vi "GetSop.vi"(8 "error in (no error)":errorcluster, 11 "ModbusSp in":refnum<class "ModbusSp.lvclass">) -> (0 "error out":errorcluster, 2 "value":bool, 3 "ModbusSp out":refnum<class "ModbusSp.lvclass">)   [LabVIEW 2019, in "ModbusSp.lvclass"]
uses:
  ModbusSp.lvclass
  ModbusSp.lvclass/ModbusSp.ctl
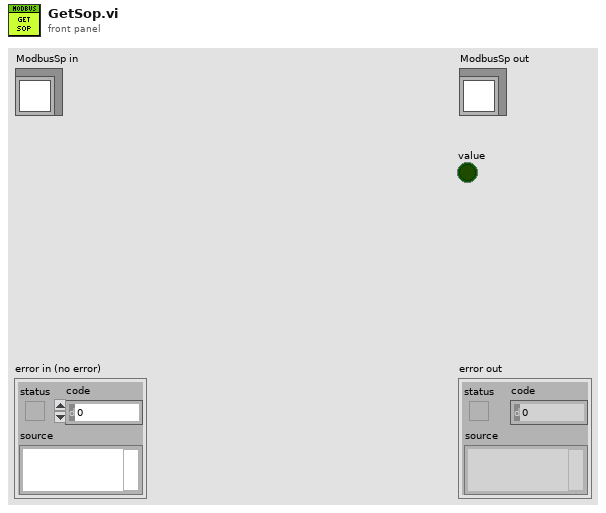
[diagram p1: front panel]
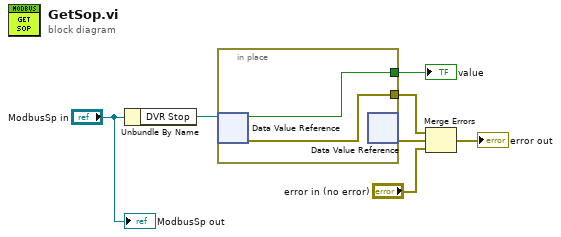
[diagram p0: block diagram]
diagram:
  n1 = Unbundle By Name("ModbusSp in") -> ("DVR Stop"=w5:refnum<data-value>)
  n2 = in-place {
    in-place-border: [w9] -> w2
    in-place-border: [w8] -> w1
    n3 = in-place-dvr #1(w5) -> (w8:bool, w9:errorcluster)
    n4 = in-place-dvr #1() -> (w3:errorcluster)  [unwired: 1 in, 1 out]
  }
  "value" <- w1
  n5 = Merge Errors(w2, w3, "error in (no error)") -> (→"error out":errorcluster)
  "ModbusSp out" <- "ModbusSp in"
